vi "Tempo.vi"   [LabVIEW 2016, in "Test2.lvrbt"]
uses:
  Test2.lvrbt
  <vilib>/NXT/Block Support/NXT_InputPort.ctl
  <vilib>/NXT/Hardware/Plugins/Tetrix 180 deg Servo/Tetrix180ServoAddress.ctl
  <vilib>/NXT/Hardware/Plugins/Tetrix DC Motor/TetrixDCMotorAddress.ctl
  <vilib>/NXT/NXTIO Xnodes/NXTIONodeSubVIs/TETRIX IO Move Servos.vi
  <vilib>/NXT/Dual Mode Library/Waits/Wait_Num.vi
  <vilib>/NXT/NXTIO Xnodes/NXTIONodeSubVIs/TETRIX IO Move DC Motors.vi
  <vilib>/NXT/Dual Mode Library/Waits/Wait_EV3_Ultrasonic_Centimeters_Further.vi
  <vilib>/NXT/NXTIO Xnodes/NXTIONodeSubVIs/TETRIX IO Stop DC Motors.vi
  <vilib>/NXT/Dual Mode Library/Waits/Wait_EV3_Ultrasonic_Centimeter_Closer.vi
  <vilib>/NXT/Subs/LVHSConnector.ctl
  <vilib>/NXT/NXTIO Xnodes/AddressXNode/NXTIOAddress.xnode
  <vilib>/NXT/NXTIO Xnodes/NXTIOXNode/NXTIO.xnode
  <vilib>/NXT/LegoClasses/BrickReference/BrickReference.lvclass
types:
  T1 = typedef "NXT_InputPort.ctl" = u32
  T2 = typedef "Tetrix180ServoAddress.ctl" = i32
  T3 = cluster{"Tetrix180Servo":T2, "Tetrix180Servo":T2, "Tetrix180Servo":T2, "Tetrix180Servo":T2}
  T4 = typedef "LVHSConnector.ctl" = refnum<class "BrickReference.lvclass">
  T5 = typedef "TetrixDCMotorAddress.ctl" = i32
  T6 = cluster{"TetrixDCMotor":T5, "TetrixDCMotor 2":T5}
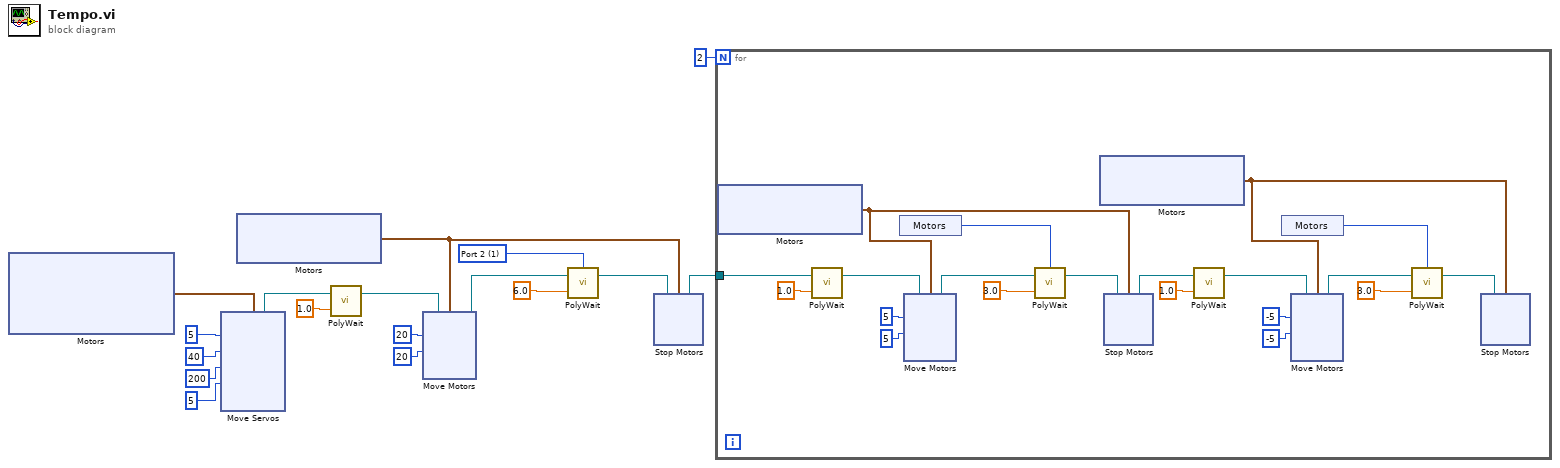
[diagram p0: block diagram]
diagram:
  w6 = T1 1 items=["Port 1", "Port 2", "Port 3", "Port 4"] ("Port (Port 1)")
  n1 = xnode "Motors"() -> ("Motor"=w17:T3)
  n2 = xnode "Move Servos"("Position 4"=u8 5, "Position 3"=u8 200, "Position 2"=u8 40, "Position 1"=u8 5, "Motors"=w17) -> ("NXT/EV3"=w12:T4)  [unwired: 1 in]
  n3 = xnode "Motors"() -> ("Motor"=w2:cluster{"TetrixDCMotor":T5, "TetrixDCMotor":T5})
  n4 = call-poly <vilib>:"PolyWait.vi"("Time (1 sec)"=sgl 1.0, "NXT/EV3"=w12) -> ("NXT/EV3"=w3:T4)  [unwired: 2 in]
  n5 = xnode "Move Motors"("Power/Speed 2"=i8 20, "Power/Speed 1"=i8 20, "Motors"=w2, "NXT/EV3"=w3) -> ("NXT/EV3"=w10:T4)
  n6 = call-poly <vilib>:"PolyWait.vi"("Centimeters (50)"=sgl 6.0, "NXT/EV3"=w10, "Port (Port 1)"=w6) -> ("NXT/EV3"=w8:T4)  [unwired: 1 in]
  n7 = xnode "Stop Motors"("Motors"=w2, "NXT/EV3"=w8) -> ("NXT/EV3"=w7:T4)
  n8 = for {
    N: 2 -> [_]
    tunnel: w7 -> [w19]
    n9 = xnode "Motors"() -> ("Motor"=w34:cluster{"TetrixDCMotor":T5, "TetrixDCMotor":T5})
    n10 = call-poly <vilib>:"PolyWait.vi"("Time (1 sec)"=sgl 1.0, "NXT/EV3"=w19) -> ("NXT/EV3"=w18:T4)  [unwired: 2 in]
    n11 = xnode "Motors"() -> ("Sensor"=w22:T1)
    n12 = xnode "Move Motors"("Power/Speed 2"=i8 5, "Power/Speed 1"=i8 5, "Motors"=w34, "NXT/EV3"=w18) -> ("NXT/EV3"=w36:T4)
    n13 = call-poly <vilib>:"PolyWait.vi"("Centimeters (40)"=sgl 3.0 ("Centimeters (50)"), "NXT/EV3"=w36, "Port (Port 1)"=w22) -> ("NXT/EV3"=w35:T4)  [unwired: 1 in]
    n14 = xnode "Motors"() -> ("Motor"=w26:cluster{"TetrixDCMotor":T5, "TetrixDCMotor":T5})
    n15 = xnode "Stop Motors"("Motors"=w34, "NXT/EV3"=w35) -> ("NXT/EV3"=w30:T4)
    n16 = call-poly <vilib>:"PolyWait.vi"("Time (1 sec)"=sgl 1.0, "NXT/EV3"=w30) -> ("NXT/EV3"=w23:T4)  [unwired: 2 in]
    n17 = xnode "Motors"() -> ("Sensor"=w21:T1)
    n18 = xnode "Move Motors"("Power/Speed 2"=i8 -5, "Power/Speed 1"=i8 -5, "Motors"=w26, "NXT/EV3"=w23) -> ("NXT/EV3"=w28:T4)
    n19 = call-poly <vilib>:"PolyWait.vi"("Centimeters (50)"=sgl 3.0, "NXT/EV3"=w28, "Port (Port 1)"=w21) -> ("NXT/EV3"=w27:T4)  [unwired: 1 in]
    n20 = xnode "Stop Motors"("Motors"=w26, "NXT/EV3"=w27) -> ()  [unwired: 1 out]
  }
